vi "findgrat.vi"(1 "Present Wavelength":dbl format="%.2f") -> (0 "Grating":i32=1 min=1 max=2 step=1)   [LabVIEW 2017]
doc: "Returns the grating position for the Present Wavelength parameter.\nUses the Globals \"Grat Wave Table\" and \"Grat Position Table\""
uses:
  m_globals.vi
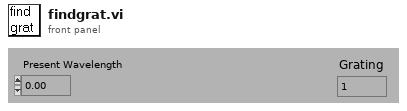
[diagram p1: front panel]
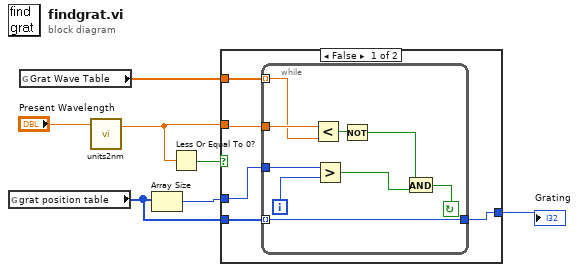
[diagram p0: block diagram]
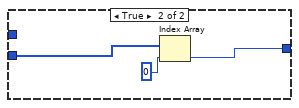
[diagram p2: hidden frame]
diagram:
  n1 = global read "m_globals.vi" "grat position table"() -> (w2:u16[])
  n2 = global read "m_globals.vi" "Grat Wave Table"() -> (w5:dbl[])
  n3 = call "units2nm.vi"("Wavelength units"="Present Wavelength") -> ("Wavelength nm"=w3:dbl)  [unwired: 1 out]
  n4 = Array Size(array=w2) -> (size(s)=w6:i32)
  n5 = Less Or Equal To 0?(x=w3) -> (x <= 0?=w7:bool)
  n6 = case shown="False" w7 {
    tunnel: w3 -> [w12 _]
    tunnel: w6 -> [w10 _]
    tunnel: w5 -> [w11 _]
    tunnel: w2 -> [w9 w22]
    tunnel: [w8 w23] -> w1
    frame False {
      n7 = while {
        tunnel: [w13] -> w8
        tunnel: w9 -> [w13] mode=indexing
        tunnel: w10 -> [w16]
        tunnel: w11 -> [w20] mode=indexing
        tunnel: w12 -> [w21]
        i -> [w15]
        stop <- w19 continue-if-true
        n8 = Less?(x=w21, y=w20) -> (x < y?=w18:bool)
        n9 = Greater?(x=w16, y=w15) -> (0:w14:bool)
        n10 = Not(x=w18) -> (.not. x?=w17:bool)
        n11 = And(x=w17, y=w14) -> (x .and. y?=w19:bool)
      }
    }
    frame True {
      n12 = Index Array(array=w22, index=0) -> (element=w23:u16)
    }
  }
  "Grating" <- w1
